vi "get_chan.vi"(11 "AI Select In":u8 format="%08b") -> (1 "Stop Loop":bool, 2 "Current Channel":u8, 3 "AI Select Out":u8)   [LabVIEW 2021]
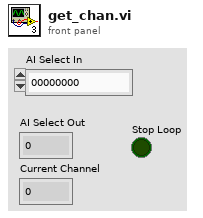
[diagram p1: front panel]
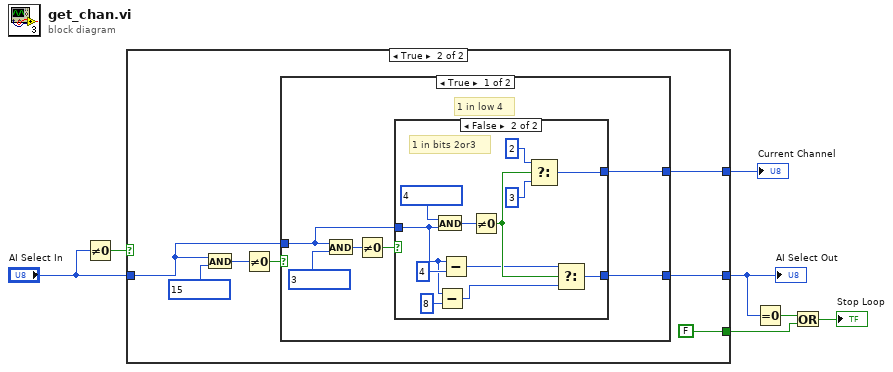
[diagram p0: block diagram]
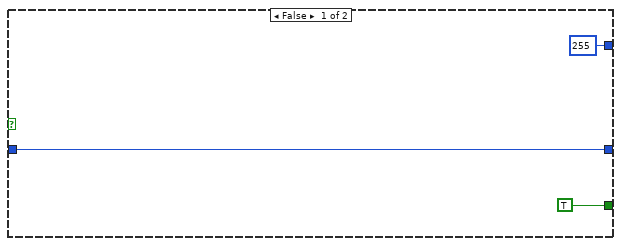
[diagram p2: hidden frame]
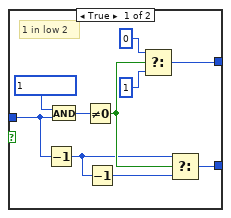
[diagram p3: hidden frame]
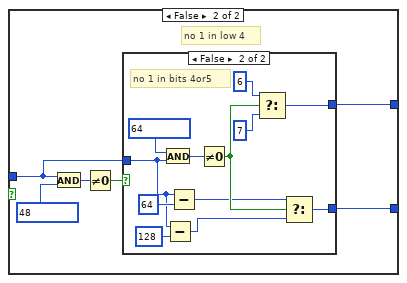
[diagram p4: hidden frame]
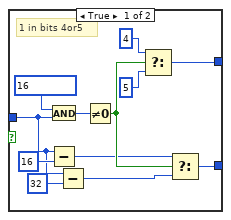
[diagram p5: hidden frame]
diagram:
  n1 = Not Equal To 0?(x="AI Select In") -> (x != 0?=w7:bool)
  n2 = case shown="True" w7 {
    tunnel: "AI Select In" -> [w9 w14]
    tunnel: [u8 255 w13] -> w2
    tunnel: [w9 w12] -> w4
    tunnel: [TRUE FALSE] -> w6
    frame False {
    }
    frame True {
      n3 = And(x=w14, y=u8 15) -> (x .and. y?=w16:u8)
      n4 = Not Equal To 0?(x=w16) -> (x != 0?=w15:bool)
      n5 = case shown="True" w15 {
        tunnel: w14 -> [w20 w48]
        tunnel: [w19 w47] -> w13
        tunnel: [w18 w46] -> w12
        frame True {
          # "1 in low 4"
          n6 = And(x=w20, y=u8 3) -> (x .and. y?=w22:u8)
          n7 = Not Equal To 0?(x=w22) -> (x != 0?=w21:bool)
          n8 = case shown="False" w21 {
            tunnel: w20 -> [w27 w36]
            tunnel: [w29 w41] -> w19
            tunnel: [w24 w39] -> w18
            frame True {
              # "1 in low 2"
              n9 = Decrement(x=w27) -> (x-1=w26:u8)
              n10 = And(x=u8 1 ("y"), y=w27) -> (x .and. y?=w32:u8)
              n11 = Not Equal To 0?(x=w32) -> (x != 0?=w28:bool)
              n12 = Decrement(x=w26) -> (x-1=w25:u8)
              n13 = Select(t=u8 0, s=w28, f=u8 1) -> (s? t:f=w29:u8)
              n14 = Select(t=w26, s=w28, f=w25) -> (s? t:f=w24:u8)
            }
            frame False {
              # "1 in bits 2or3"
              n15 = And(x=u8 4 ("y"), y=w36) -> (x .and. y?=w44:u8)
              n16 = Subtract(x=w36, y=u8 8) -> (x-y=w34:u8)
              n17 = Subtract(x=w36, y=u8 4) -> (x-y=w38:u8)
              n18 = Not Equal To 0?(x=w44) -> (x != 0?=w40:bool)
              n19 = Select(t=u8 2, s=w40, f=u8 3) -> (s? t:f=w41:u8)
              n20 = Select(t=w38, s=w40, f=w34) -> (s? t:f=w39:u8)
            }
          }
        }
        frame False {
          # "no 1 in low 4"
          n21 = And(x=w48, y=u8 48) -> (x .and. y?=w50:u8)
          n22 = Not Equal To 0?(x=w50) -> (x != 0?=w49:bool)
          n23 = case shown="False" w49 {
            tunnel: w48 -> [w54 w66]
            tunnel: [w59 w71] -> w47
            tunnel: [w57 w69] -> w46
            frame True {
              # "1 in bits 4or5"
              n24 = And(x=u8 16 ("y"), y=w54) -> (x .and. y?=w62:u8)
              n25 = Subtract(x=w54, y=u8 16) -> (x-y=w55:u8)
              n26 = Subtract(x=w54, y=u8 32) -> (x-y=w52:u8)
              n27 = Not Equal To 0?(x=w62) -> (x != 0?=w58:bool)
              n28 = Select(t=u8 4, s=w58, f=u8 5) -> (s? t:f=w59:u8)
              n29 = Select(t=w55, s=w58, f=w52) -> (s? t:f=w57:u8)
            }
            frame False {
              # "no 1 in bits 4or5"
              n30 = And(x=u8 64 ("y"), y=w66) -> (x .and. y?=w74:u8)
              n31 = Subtract(x=w66, y=u8 128) -> (x-y=w64:u8)
              n32 = Subtract(x=w66, y=u8 64) -> (x-y=w68:u8)
              n33 = Not Equal To 0?(x=w74) -> (x != 0?=w70:bool)
              n34 = Select(t=u8 6, s=w70, f=u8 7) -> (s? t:f=w71:u8)
              n35 = Select(t=w68, s=w70, f=w64) -> (s? t:f=w69:u8)
            }
          }
        }
      }
    }
  }
  "AI Select Out" <- w4
  "Current Channel" <- w2
  n36 = Equal To 0?(x=w4) -> (x = 0?=w5:bool)
  n37 = Or(x=w5, y=w6) -> (x .or. y?=→"Stop Loop":bool)
